vi "HandleAlarms.vi"(0 "reference in":refnum<class "Sig_AI.lvclass">, 11 "error in (no error)":errorcluster) -> (4 "reference out":refnum<class "Sig_AI.lvclass">, 15 "error out":errorcluster)   [LabVIEW 2019, in "Sig_AI.lvclass"]
uses:
  Sig_AI.lvclass
  Sig_AI.lvclass/Sig_AI.ctl
  AnalogComparator_class/AnalogComparator.lvclass/AnalogComparator.ctl
  AnalogComparator_class/HandleDb.vi
  AnalogComparator_class/AnalogComparator.lvclass
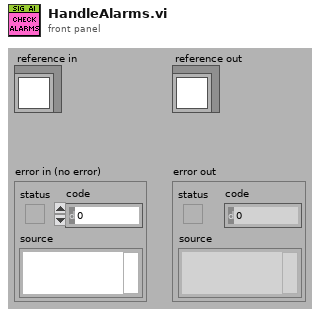
[diagram p1: front panel]
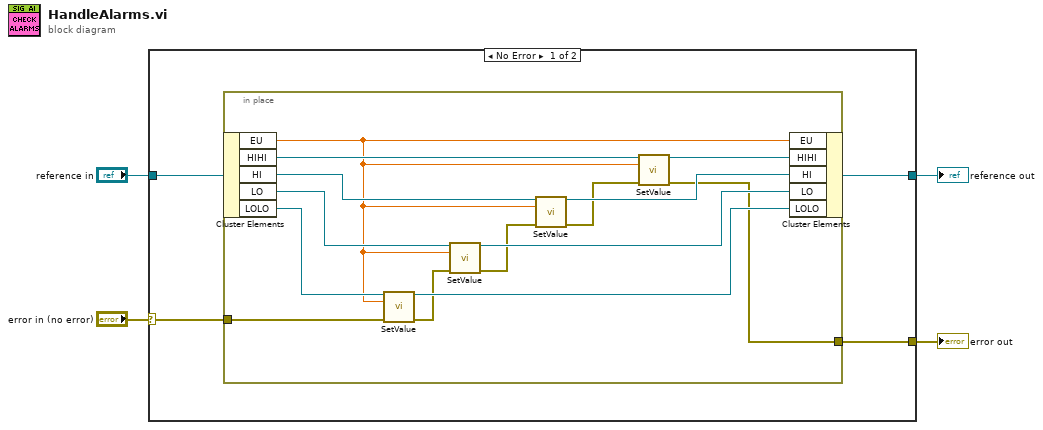
[diagram p0: block diagram]
diagram:
  n1 = case shown="No Error" "error in (no error)" {
    selector: "error in (no error)" -> [w5 w24]
    tunnel: [w6 w24] -> w3
    tunnel: [w7 w23] -> w1
    tunnel: "reference in" -> [w8 w23]
    frame No Error {
      n2 = in-place {
        in-place-border: [w10] -> w6
        in-place-border: w5 -> [w9]
        n3 = in-place-cluster #1(w8) -> ("EU"=w14:dbl, "HIHI"=w22:refnum<class "AnalogComparator.lvclass">, "HI"=w20:refnum<class "AnalogComparator.lvclass">, "LO"=w18:refnum<class "AnalogComparator.lvclass">, "LOLO"=w16:refnum<class "AnalogComparator.lvclass">)
        n4 = call "SetValue.vi"("class data in"=w16, "Value"=w14, "error in (no error)"=w9) -> ("class data out"=w15:refnum<class "AnalogComparator.lvclass">, "error out"=w13:errorcluster)  [unwired: 11 in]
        n5 = call "SetValue.vi"("class data in"=w18, "Value"=w14, "error in (no error)"=w13) -> ("class data out"=w17:refnum<class "AnalogComparator.lvclass">, "error out"=w12:errorcluster)  [unwired: 11 in]
        n6 = call "SetValue.vi"("class data in"=w20, "Value"=w14, "error in (no error)"=w12) -> ("class data out"=w19:refnum<class "AnalogComparator.lvclass">, "error out"=w11:errorcluster)  [unwired: 11 in]
        n7 = call "SetValue.vi"("class data in"=w22, "Value"=w14, "error in (no error)"=w11) -> ("class data out"=w21:refnum<class "AnalogComparator.lvclass">, "error out"=w10:errorcluster)  [unwired: 11 in]
        n8 = in-place-cluster #1("EU"=w14, "HIHI"=w21, "HI"=w19, "LO"=w17, "LOLO"=w15) -> (w7:refnum<class "Sig_AI.lvclass">)
      }
    }
    frame Error {
    }
  }
  "error out" <- w3
  "reference out" <- w1
